vi "file zip.vi"() -> ()   [LabVIEW 2013]
panel:
  out "appended path":path
  in  "path":path
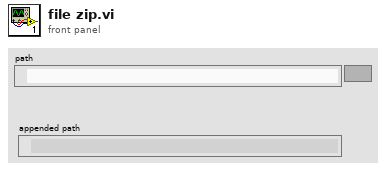
[diagram p1: front panel]
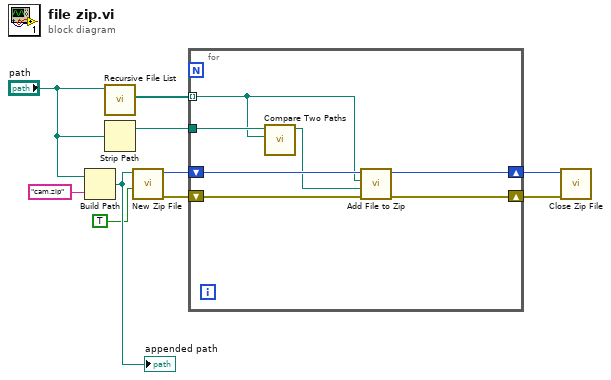
[diagram p0: block diagram]
diagram:
  n1 = Build Path(base path="path", name or relative path="cam.zip") -> (appended path=w9:path)
  "appended path" <- w9
  n2 = call <vilib>:"Recursive File List.vi"("Folder Path"="path") -> ("All Files in Dir"=w3:path[])  [unwired: 6 in, 4 out]
  n3 = Strip Path(path="path") -> (stripped path=w1:path)  [unwired: 1 out]
  n4 = call <vilib>:"New Zip File.vi"("confirm overwrite? (F)"=TRUE, "target"=w9) -> ("error out"=w6:errorcluster, "zip file out"=w7:i64)  [unwired: 3 in, 1 out]
  n5 = for {
    shift-right: [w16] -> w5
    shift-left: w7 -> [w17]
    shift-right: [w14] -> w4
    shift-left: w6 -> [w15]
    tunnel: w3 -> [w12] mode=indexing
    tunnel: w1 -> [w13]
    n6 = call <vilib>:"Compare Two Paths.vi"("Path 2"=w12, "Path 1"=w13) -> ("Relative Path from 1 to 2"=w11:path)  [unwired: 6 in, 3 out]
    n7 = call <vilib>:"Add File to Zip.vi"("error in (no error)"=w15, "destination path in zip"=w11, "source file path"=w12, "zip file in"=w17) -> ("error out"=w14:errorcluster, "zip file out"=w16:i64)  [unwired: 6 in]
  }
  n8 = call <vilib>:"Close Zip File.vi"("error in (no error)"=w4, "zip file in"=w5) -> ()  [unwired: 5 in, 1 out]
